vi "Reply.vi"(7 "Original Payload":T1, 8 "error in (no error)":errorcluster, 9 "Type":string, 10 "Payload":u8[](array[numeric]), 11 "TCPMessageAPI in":refnum<class "TCPMessageAPI.lvclass">) -> (0 "error out":errorcluster, 3 "TCPMessageAPI out":refnum<class "TCPMessageAPI.lvclass">)   [LabVIEW 2020, in "Vecto.lvlib" / "TCPMessageAPI.lvclass"]
uses:
  TCPMessageAPI.lvclass
  lv-volatus/messages/TcpPayload/Data.ctl
  lv-volatus/messages/TcpReply/Data.ctl
  TCPMessageAPI.lvclass/TCPMessageAPI.ctl
  lv-volatus/messages/TcpReply/TcpReply.lvlib
  lv-volatus/messages/TcpPayload/TcpPayload.lvlib
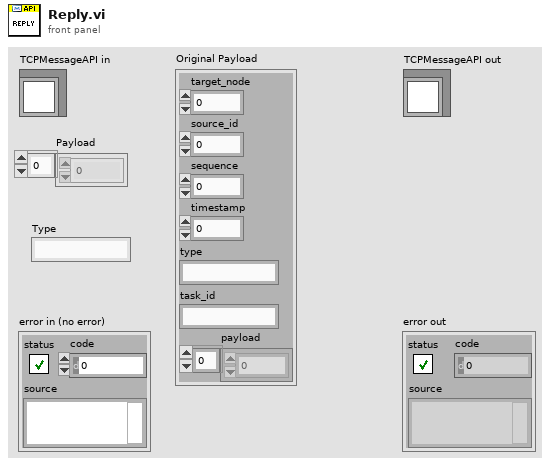
[diagram p1: front panel]
types:
  T1 = typedef "TcpPayload.lvlib/Data.ctl" = cluster{"target_node":u32, "source_id":u32, "sequence":u32, "timestamp":i64, "type":string, "task_id":string, "payload":u8[]}
  T2 = typedef "TcpReply.lvlib/Data.ctl" = cluster{"request_sequence":u32, "request_timestamp":u64, "payload":u8[], "type":string}
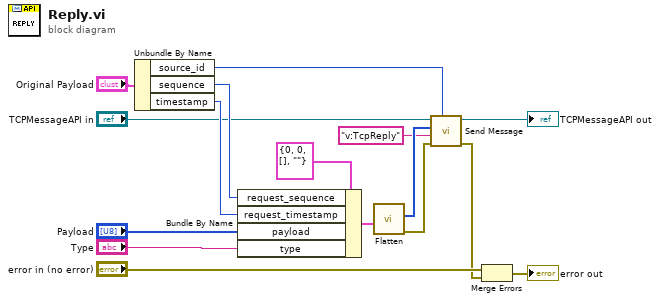
[diagram p0: block diagram]
diagram:
  n1 = Unbundle By Name("Original Payload") -> ("source_id"=w5:u32, "sequence"=w12:u32, "timestamp"=w11:i64)
  n2 = Bundle By Name(cluster=T2 {"request_sequence"=0, "request_timestamp"=0, "payload"=[], "type"=""} ("TcpReply"), "request_sequence"=w12, "request_timestamp"=w11, "payload"="Payload", "type"="Type") -> (w10:T2)
  n3 = call "Flatten.vi"("Data"=w10) -> ("error out"=w6:errorcluster, "Buffer"=w7:u8[])  [unwired: 9 in]
  n4 = call "Send Message.vi"("Target ID"=w5, "error in (no error)"=w6, "Type"="v:TcpReply" ("TcpReply"), "Payload"=w7, "TCPMessageService in"="TCPMessageAPI in") -> ("error out"=w3:errorcluster, "TCPMessageService out"=→"TCPMessageAPI out":refnum<class "TCPMessageAPI.lvclass">)  [unwired: 5 in]
  n5 = Merge Errors("error in (no error)", w3) -> (→"error out":errorcluster)
